vi "coords_add.vi"(8 "DEC 2 (arcsec)":dbl format="%<%H:%M:%S%1u>t", 9 "DEC 1 (arcsec)":dbl format="%<%H:%M:%S>t", 10 "RA 2 (arcsec)":dbl format="%<%H:%M:%S%1u>t", 11 "RA 1 (arcsec)":dbl format="%<%H:%M:%S%1u>t") -> (0 "DEC OUT":dbl format="%<%H:%M:%S%1u>t", 1 "DEC OUT (deg)":dbl format="%.3f", 2 "RA OUT (deg)":dbl format="%.3f", 3 "RA OUT":dbl format="%<%H:%M:%S%1u>t")   [LabVIEW 2010]
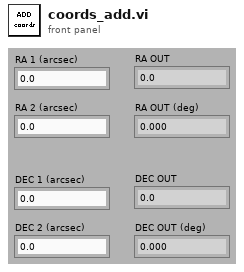
[diagram p1: front panel]
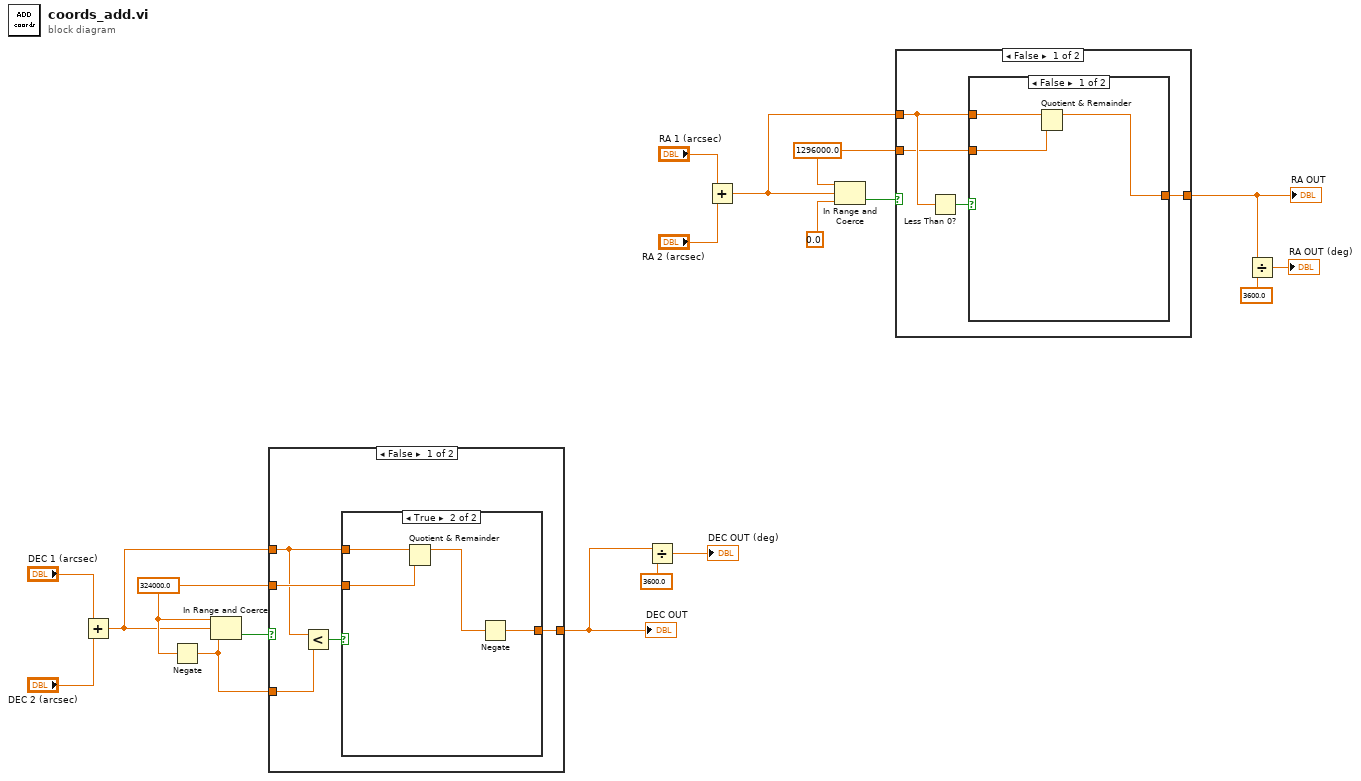
[diagram p0: block diagram]
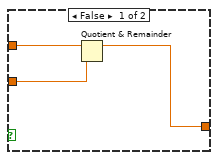
[diagram p2: hidden frame]
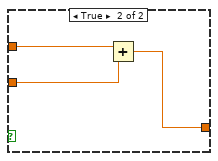
[diagram p4: hidden frame]
diagram:
  w9 = 324000.0
  w13 = 1296000.0
  n1 = Add(x="DEC 1 (arcsec)", y="DEC 2 (arcsec)") -> (x+y=w7:dbl)
  n2 = Negate(x=w9) -> (-x=w8:dbl)
  n3 = In Range and Coerce(upper limit=w9, x=w7, lower limit=w8) -> (In Range?=w11:bool)  [unwired: 1 out]
  n4 = case shown="False" w11 {
    tunnel: w7 -> [w20 w31]
    tunnel: [w22 w31] -> w6
    tunnel: w9 -> [w21 _]
    tunnel: w8 -> [w19 _]
    frame False {
      n5 = Less?(x=w20, y=w19) -> (x < y?=w23:bool)
      n6 = case shown="True" w23 {
        tunnel: w20 -> [w26 w30]
        tunnel: [w24 w27] -> w22
        tunnel: w21 -> [w25 w29]
        frame False {
          n7 = Quotient & Remainder(x=w26, y=w25) -> (x-y*floor(x/y)=w24:dbl)  [unwired: 1 out]
        }
        frame True {
          n8 = Quotient & Remainder(x=w30, y=w29) -> (x-y*floor(x/y)=w28:dbl)  [unwired: 1 out]
          n9 = Negate(x=w28) -> (-x=w27:dbl)
        }
      }
    }
    frame True {
    }
  }
  "DEC OUT" <- w6
  n10 = Divide(x=w6, y=3600.0) -> (x/y=→"DEC OUT (deg)":dbl)
  n11 = Add(x="RA 1 (arcsec)", y="RA 2 (arcsec)") -> (x+y=w14:dbl)
  n12 = In Range and Coerce(upper limit=w13, x=w14, lower limit=0.0) -> (In Range?=w15:bool)  [unwired: 1 out]
  n13 = case shown="False" w15 {
    tunnel: w14 -> [w34 w42]
    tunnel: [w33 w42] -> w1
    tunnel: w13 -> [w32 _]
    frame False {
      n14 = Less Than 0?(x=w34) -> (x < 0?=w35:bool)
      n15 = case shown="False" w35 {
        tunnel: w34 -> [w38 w41]
        tunnel: [w36 w40] -> w33
        tunnel: w32 -> [w37 w39]
        frame False {
          n16 = Quotient & Remainder(x=w38, y=w37) -> (x-y*floor(x/y)=w36:dbl)  [unwired: 1 out]
        }
        frame True {
          n17 = Add(x=w41, y=w39) -> (x+y=w40:dbl)
        }
      }
    }
    frame True {
    }
  }
  "RA OUT" <- w1
  n18 = Divide(x=w1, y=3600.0) -> (x/y=→"RA OUT (deg)":dbl)
